vi "Configure Auto IF Bandwidth.vi"(7 "Enable Auto IF Bandwidth (T: Enable)":bool=TRUE, 8 "error in (no error)":errorcluster, 9 "Max Bandwidth Limit (3E4)":dbl=30000.0, 10 "Active Channel (1)":i32=1, 11 "VISA resource name":refnum<visa-resource-name>) -> (0 "error out":errorcluster, 3 "VISA resource name out":refnum<visa-resource-name>)   [LabVIEW 2022 SP3, in "Agilent ENA Series.lvlib"]
doc: "Configures IF Bandwidth auto function.\n\n<B>Note:</B> This VI is only valid for E5061B."
uses:
  <instrlib>/Agilent ENA Series/Agilent ENA Series.lvlib
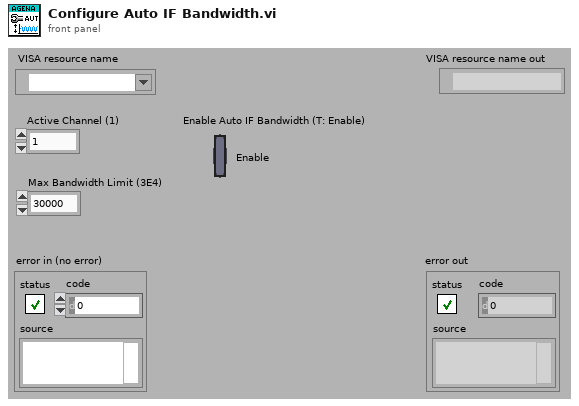
[diagram p1: front panel]
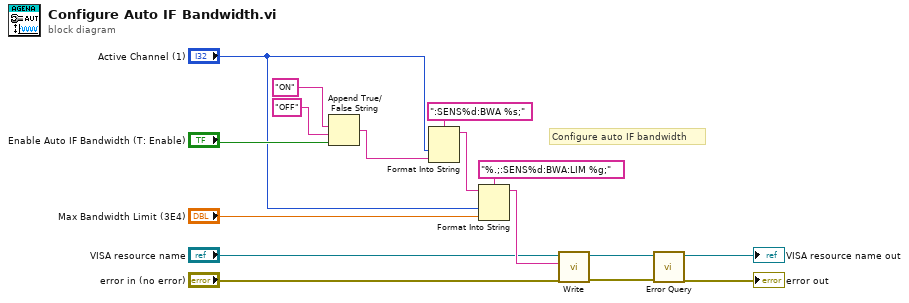
[diagram p0: block diagram]
diagram:
  # "Configure auto IF bandwidth"
  n1 = Append True/False String(1:"Enable Auto IF Bandwidth (T: Enable)", 2:"OFF", 3:"ON") -> (0:w11:string)  [unwired: 1 out]
  n2 = Format Into String(format string=":SENS%d:BWA %s;", "Active Channel (1)", w11) -> (resulting string=w10:string)  [unwired: 2 in, 1 out]
  n3 = Format Into String(format string="%.;:SENS%d:BWA:LIM %g;", initial string=w10, "Active Channel (1)", "Max Bandwidth Limit (3E4)") -> (resulting string=w5:string)  [unwired: 1 in, 1 out]
  n4 = call <instrlib>:"Write.vi"("error in (no error)"="error in (no error)", "String ()"=w5, "VISA resource name"="VISA resource name") -> ("error out"=w1:errorcluster, "VISA resource name out"=w2:refnum<visa-resource-name>)  [unwired: 6 in, 1 out]
  n5 = call <instrlib>:"Error Query.vi"("error in (no error)"=w1, "VISA resource name"=w2) -> ("error out"=→"error out":errorcluster, "VISA resource name out"=→"VISA resource name out":refnum<visa-resource-name>)  [unwired: 8 out]
